vi "GetDisplayMode.vi"(8 "Error In":errorcluster, 11 "Keithley 6482 In":refnum<visa-resource-name>) -> (0 "Error Out":errorcluster, 2 "Display Mode":T1, 3 "Keithley 6482 Out":refnum<visa-resource-name>)   [LabVIEW 2009, in "Keithley-6482-Visa.lvlib"]
uses:
  <instrlib>/Keithley-6482-Visa9.0/Keithley-6482-Visa.lvlib
  <instrlib>/Keithley-6482-Visa9.0/Public/Controls/DisplayMode.ctl
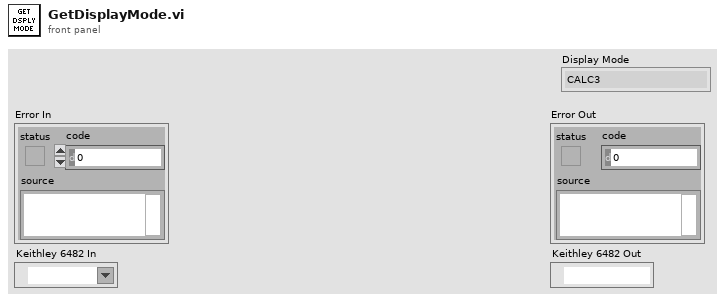
[diagram p1: front panel]
types:
  T1 = typedef "Keithley-6482-Visa.lvlib/DisplayMode.ctl" = enum16{"CALC3", "CALC4", "CALC5", "CALC6", "DUAL"}
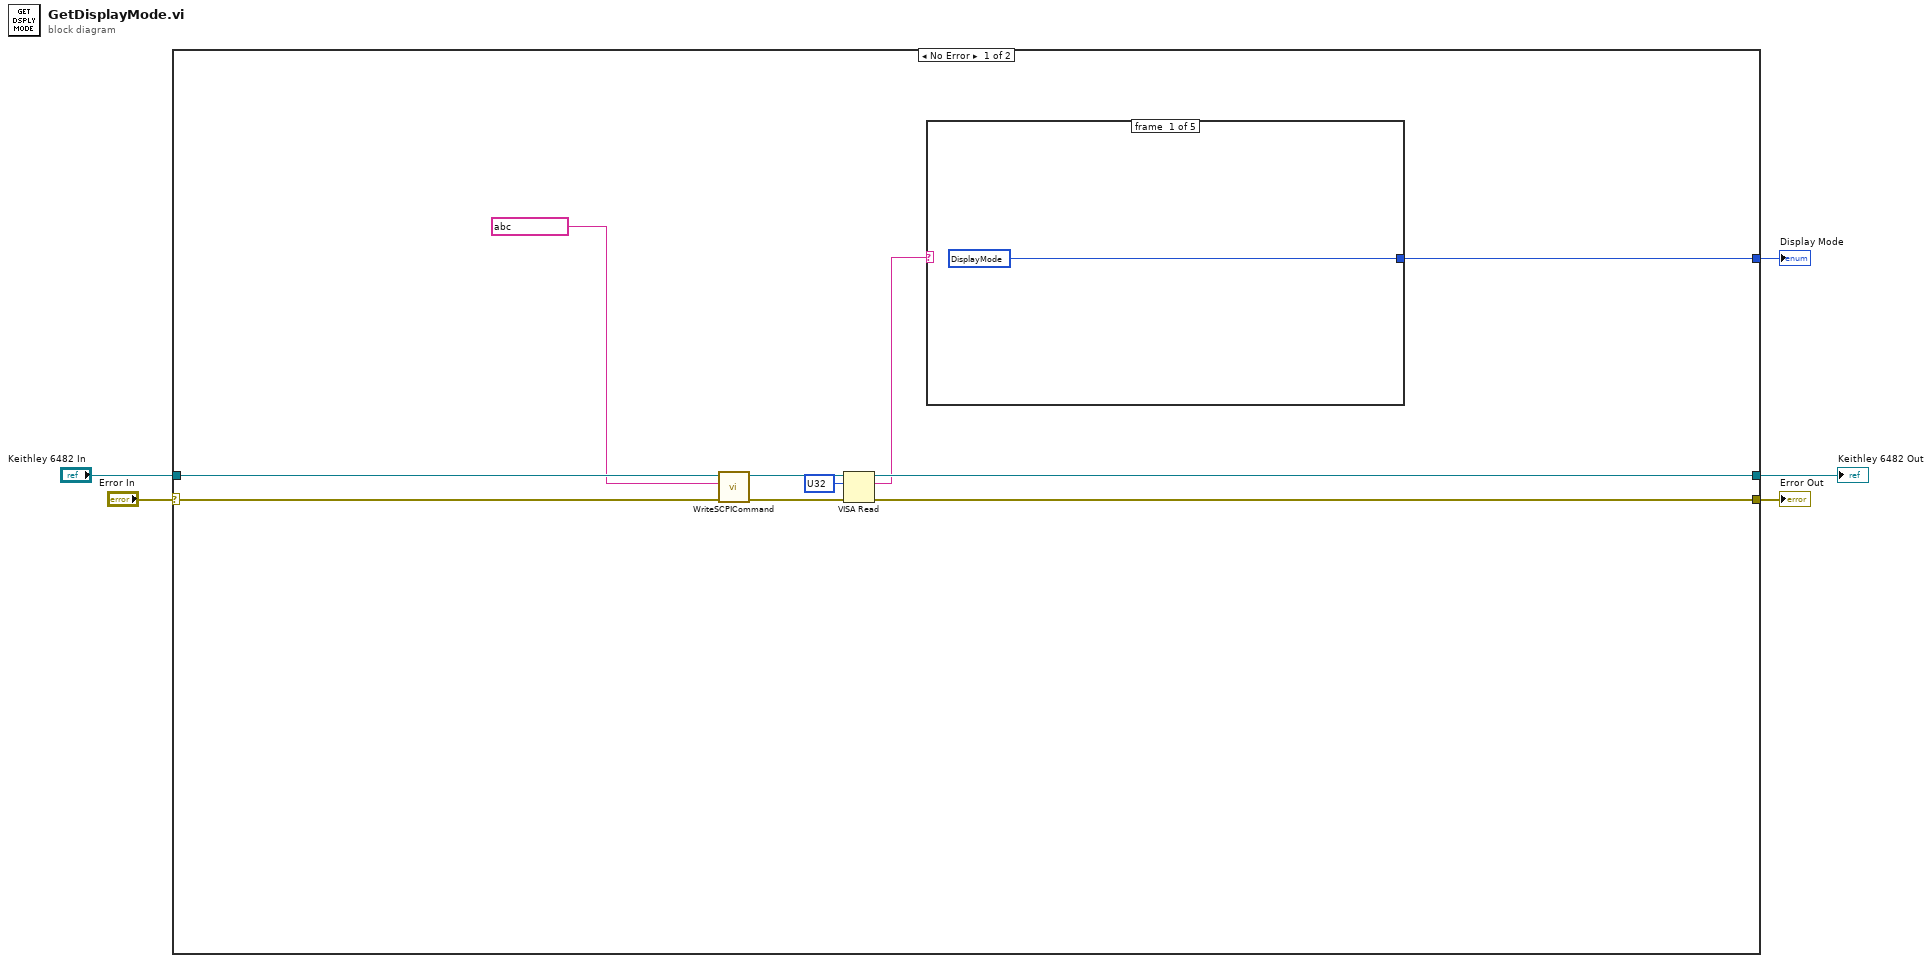
[diagram p0: block diagram]
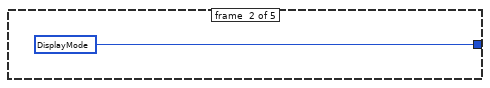
[diagram p2: hidden frame]
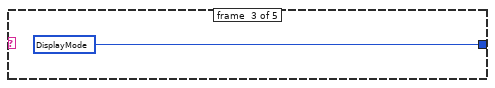
[diagram p3: hidden frame]
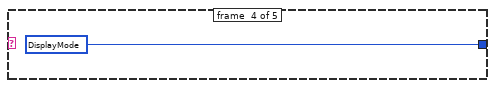
[diagram p4: hidden frame]
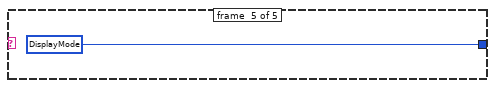
[diagram p5: hidden frame]
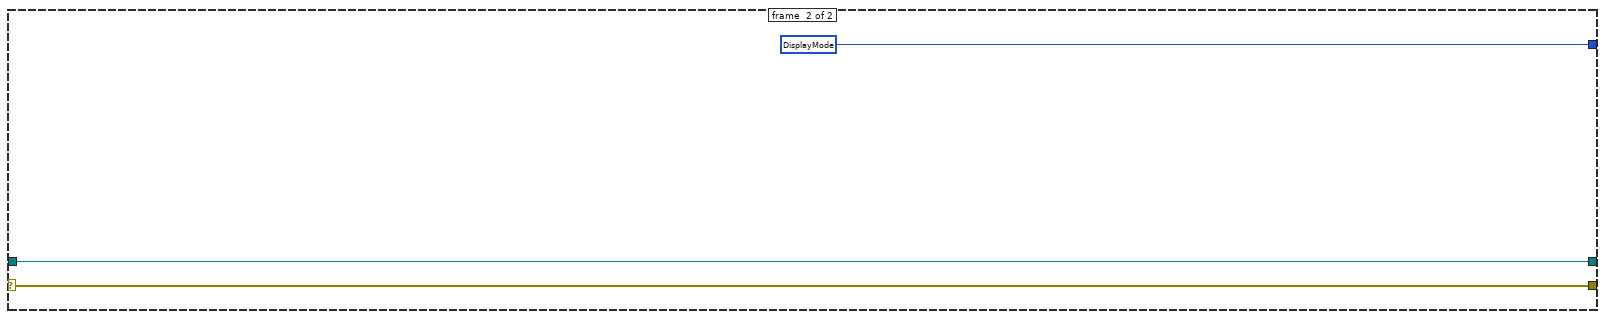
[diagram p6: hidden frame]
diagram:
  n1 = case shown="No Error" "Error In" {
    selector: "Error In" -> [w8 w22]
    tunnel: [w15 w22] -> w4
    tunnel: [w14 w23] -> w3
    tunnel: "Keithley 6482 In" -> [w7 w23]
    tunnel: [w11 T1 ? ("Display Mode")] -> w1
    frame #0 {
      n2 = call <instrlib>:"WriteSCPICommand.vi"("Error In"=w8, "SCPI Command"=string ?, "Keithley 6482 In"=w7) -> ("Error Out"=w9:errorcluster, "Keithley 6482 Out"=w10:refnum<visa-resource-name>)  [unwired: 7 in]
      n3 = VISA Read(VISA resource name=w10, byte count=u32 ?, error in (no error)=w9) -> (VISA resource name out=w14:refnum<visa-resource-name>, read buffer=w12:string, error out=w15:errorcluster)  [unwired: 1 out]
      n4 = case shown="\"DUAL\"" w12 {
        tunnel: [T1 ? ("Display Mode") T1 ? ("Display Mode") T1 ? ("Display Mode") T1 ? ("Display Mode") T1 ? ("Display Mode")] -> w11
        frame #0 {
        }
        frame #1 {
        }
        frame #2 {
        }
        frame #3 {
        }
        frame #4 {
        }
      }
    }
    frame #1 {
    }
  }
  "Error Out" <- w4
  "Keithley 6482 Out" <- w3
  "Display Mode" <- w1
